vi "Example Main Program.vi"() -> ()   [LabVIEW 2018]
uses:
  Feedback Controller Gains.ctl
  <vilib>/Platform/TimedLoop/XDataNode/timing_clust.ctl
  <vilib>/Platform/TimedLoop/XDataNode/nitl_modes.ctl
  <vilib>/Platform/TimedLoop/XDataNode/wakeup.ctl
  <vilib>/platform/TimedLoop/XDataNode/XDataNode.xnode
  <vilib>/Platform/TimedLoop/XDataNode/XDNodeRunTimeDep.lvlib
  COBRA Feedback Control Library.lvlib
panel:
  out "Motor Velocity Command (deg/s)":dbl
  out "Velocity":T1(graph)
  out "Motor Velocity (deg/s)":dbl
  out "Force":T2(graph)
  in  "Stop":bool
  out "Error (N)":dbl
  out "Force (N)":dbl
  in  "Force Setpoint (N)":dbl
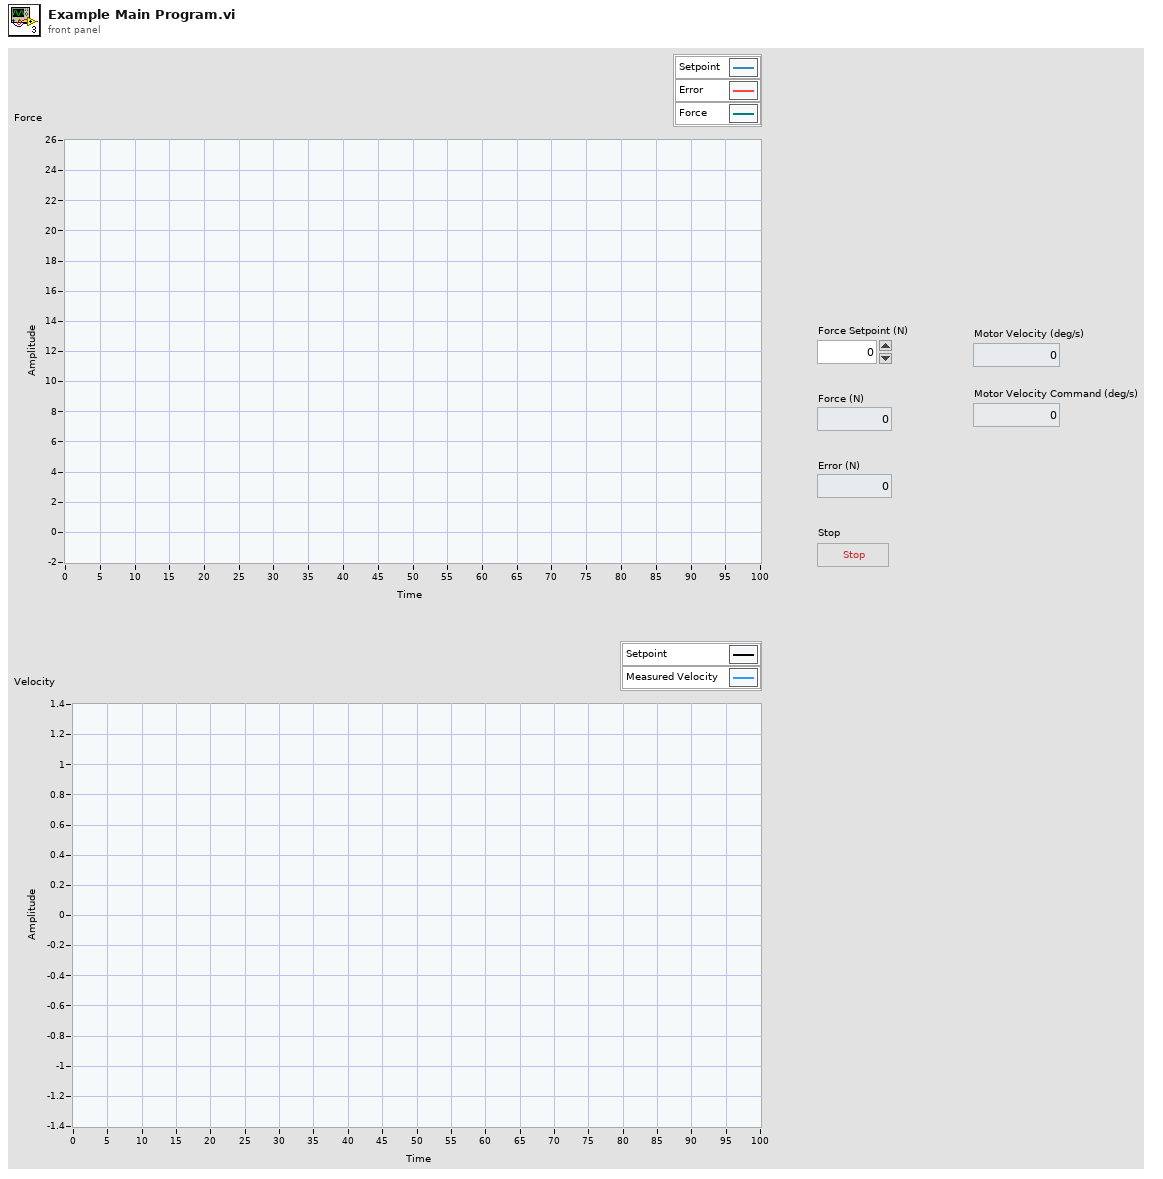
[diagram p1: front panel]
types:
  T1 = cluster{"Motor Velocity (deg/s)":dbl, "Motor Velocity Command (deg/s)":dbl}
  T2 = cluster{"Force Setpoint (N)":dbl, "Error (N)":dbl, "Force (N)":dbl}
  T3 = typedef "XDNodeRunTimeDep.lvlib/timing_clust.ctl" = cluster{"Expected End [f-1]":u64, "Actual End [f-1]":u64, "Finished Late? [f-1]":bool, "Expected End [i-1]":u64, "Actual End [i-1]":u64, "Finished Late? [i-1]":bool, "Expected Start [i]":u64, "Actual Start [i]":u64, "Expected Start [f]":u64, "Actual Start [f]":u64, "Source Name":string, "Structure Name":string, "Period":i64, "Deadline":i64, "Offset":i64, "Start":i64, "Priority":i32, "Timeout":i32, "Mode":T4, "Wakeup Reason":T5, "Error":errorcluster, "Source Type":string, "Secondary Source Type":string, "Global End Time":u64, "Global Start Time":u64, "Frame Duration":u64, "Iteration Duration":u64, "Assigned CPU":i32, "I/O Scan Engine Mode":u32}
  T4 = typedef "XDNodeRunTimeDep.lvlib/nitl_modes.ctl" = enum32{"No Change", "Process missed periods, maintain original phase", "Discard missed periods, maintain original phase", "Process missed periods, ignore original phase", "Discard missed periods, ignore original phase"}
  T5 = typedef "XDNodeRunTimeDep.lvlib/wakeup.ctl" = enum32{"Normal", "Aborted", "Asynchronous wakeup", "Timing source error", "Timed loop error", "Timeout"}
  T6 = typedef "COBRA Feedback Control Library.lvlib/Feedback Controller Gains.ctl" = cluster{"Kp":dbl, "Kd":dbl}
  T7 = cluster{"Motor Velocity Command (deg/s)":dbl, "Motor Velocity (deg/s)":dbl}
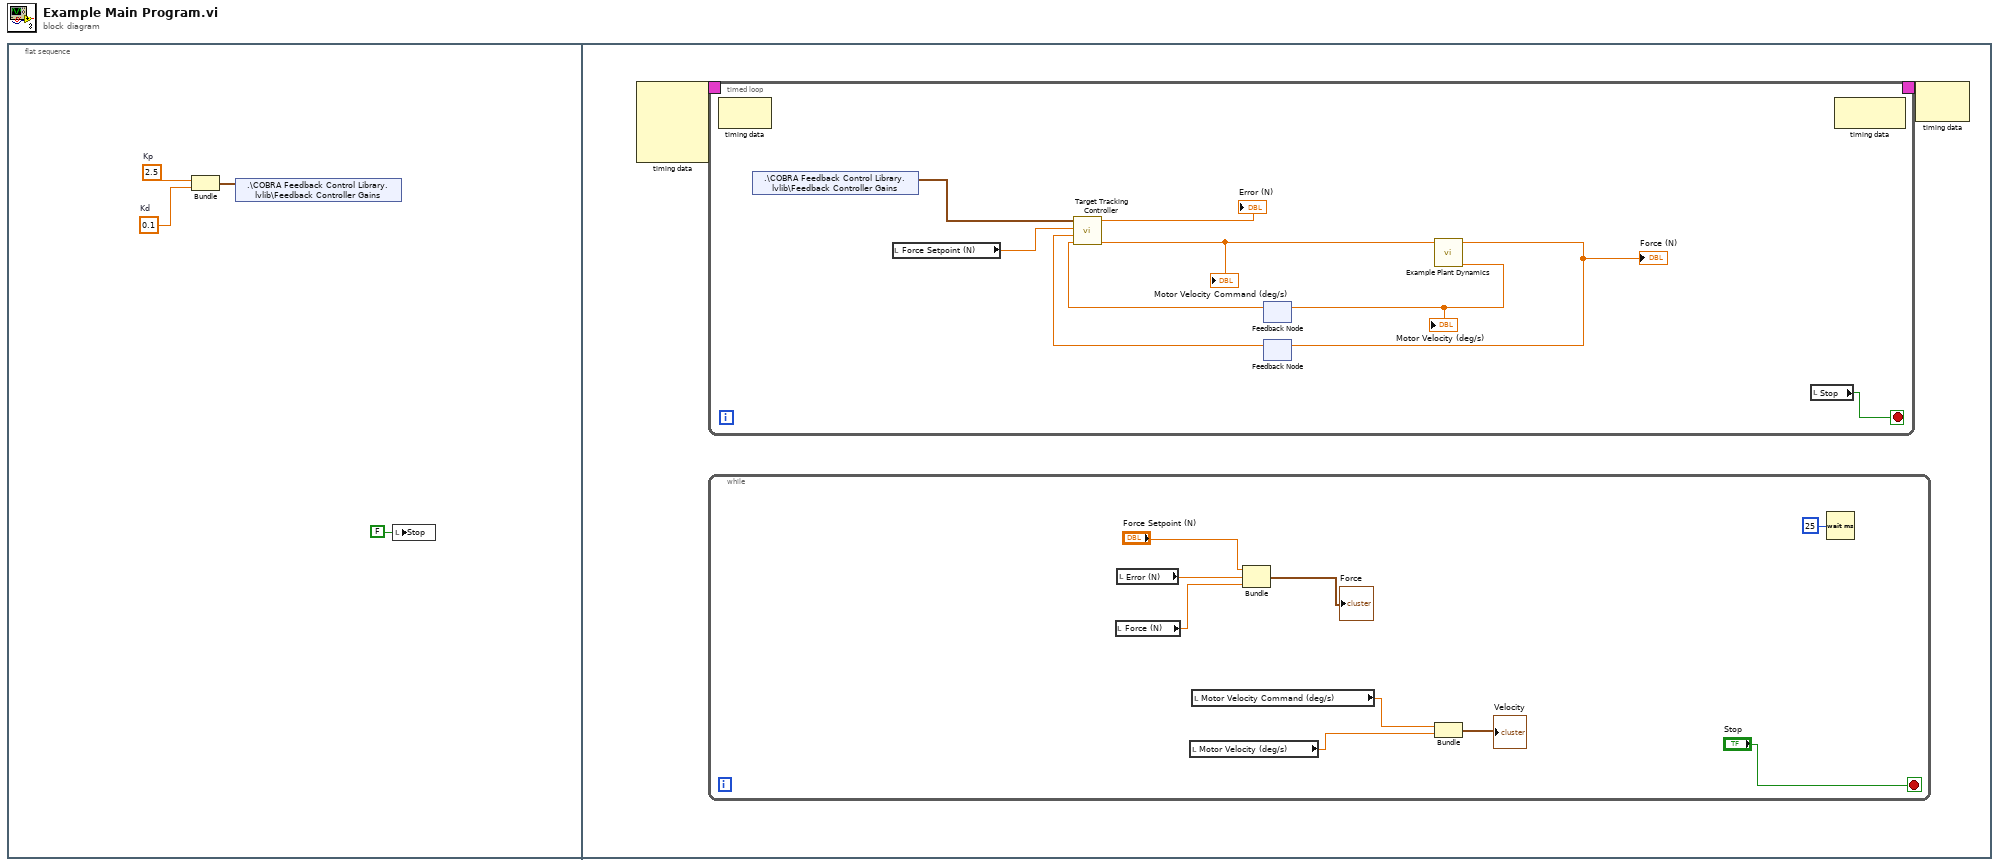
[diagram p0: block diagram]
diagram:
  n1 = flat-sequence {
    frame #0 {
      w1 = 0.1  # Kd
      w2 = 2.5  # Kp
      n2 = Bundle("Kp"=w2, "Kd"=w1) -> (w3:cluster{"Kp":dbl, "Kd":dbl})  [unwired: 1 in]
      n3 = shared-variable ".\\COBRA Feedback Control Library.lvlib\\Feedback Controller Gains"(w3) -> ()  [unwired: 1 in, 1 out]
      n4 = local write "Stop"(FALSE ("Stop")) -> ()
    }
    frame #1 {
      n5 = node-c288() -> (w6:T3)  [unwired: 4 in]
      n6 = timed-loop {
        timing: w6 -> [_]
        timing-out: [_] -> w5
        stop <- w16 stop-if-true
        n7 = node-c288() -> ()  [unwired: 1 in, 1 out]
        n8 = shared-variable ".\\COBRA Feedback Control Library.lvlib\\Feedback Controller Gains"() -> (w24:T6)  [unwired: 1 in, 1 out]
        n9 = local read "Force Setpoint (N)"() -> (w23:dbl)
        n10 = feedback #1() -> (w18:dbl)  [unwired: 1 in]
        n11 = feedback #2() -> (w22:dbl)  [unwired: 1 in]
        n12 = call "Target Tracking Controller.vi"("Motor Velocity (deg/s)"=w18, "Filtered Force (N)"=w22, "Force Setpoint (N)"=w23, "Feedback Controller Gains"=w24) -> ("Motor Velocity Command (deg/s)"=w21:dbl, "Error (N)"=→"Error (N)":dbl)  [unwired: 6 in]
        "Motor Velocity Command (deg/s)" <- w21
        n13 = call "Example Plant Dynamics.vi"("Motor Velocity Command (deg/s)"=w21) -> ("Motor Velocity (deg/s)"=w19:dbl, "Force"=w20:dbl)  [unwired: 9 in]
        "Force (N)" <- w20
        "Motor Velocity (deg/s)" <- w19
        n14 = feedback-in #1(w19) -> ()
        n15 = feedback-in #2(w20) -> ()
        n16 = local read "Stop"() -> (w16:bool)
        n17 = node-c288() -> ()  [unwired: 1 in, 1 out]
      }
      n18 = while {
        stop <- "Stop" stop-if-true
        n19 = local read "Force (N)"() -> (w11:dbl)
        n20 = local read "Error (N)"() -> (w12:dbl)
        n21 = local read "Motor Velocity (deg/s)"() -> (w9:dbl)
        n22 = local read "Motor Velocity Command (deg/s)"() -> (w8:dbl)
        n23 = Bundle("Force Setpoint (N)"="Force Setpoint (N)", "Error (N)"=w12, "Force (N)"=w11) -> (→"Force":T2)  [unwired: 1 in]
        n24 = Bundle("Motor Velocity Command (deg/s)"=w8, "Motor Velocity (deg/s)"=w9) -> (→"Velocity":T7)  [unwired: 1 in]
        n25 = Wait (ms)(milliseconds to wait=u32 25) -> ()  [unwired: 1 out]
      }
      n26 = node-c288(w5) -> ()  [unwired: 1 out]
    }
  }
